vi "SlideBoundsWrite.vi"(4 "error in (no error)":errorcluster, 5 "Value":cluster{"min":i16, "max":i16}, 6 "Container State":T2, 7 "Display State In":T1) -> (0 "error out":errorcluster, 3 "Display State Out":T1)   [LabVIEW 2019, in "XVerticalSlide.xctl"]
uses:
  XVerticalSlide.xctl
  <vilib>/_xctls/Container State.ctl
  State.ctl
  <vilib>/_xctls/XControlSupport.lvlib
panel:
  # "Replace the Value Control below with a Control of desired type.\nDo not remove this Control or the others from the connector pane.\nDo not change the connector pane pattern.\nThe Value control should always be the third terminal from top on the input side in the connector pane."
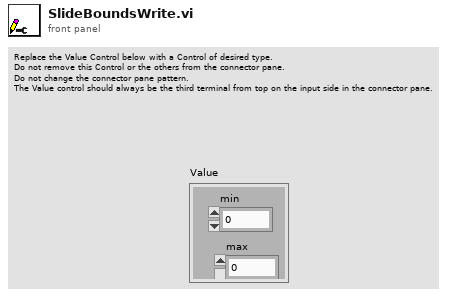
[diagram p1: front panel]
types:
  T1 = typedef "XVerticalSlide.xctl/State.ctl" = cluster{"low":i16, "high":i16, "min":i16, "max":i16}
  T2 = typedef "XControlSupport.lvlib/Container State.ctl" = cluster{"Indicator?":bool, "Run Mode?":bool, " Refnum":refnum<vi>}
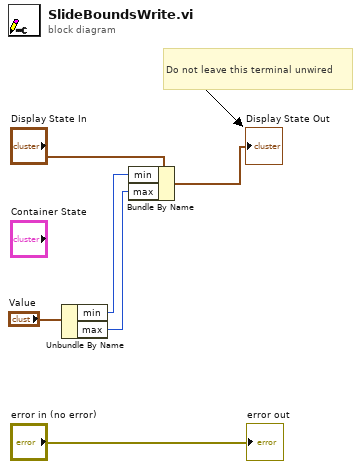
[diagram p0: block diagram]
diagram:
  # "Do not leave this terminal unwired"
  n1 = Unbundle By Name("Value") -> ("min"=w3:i16, "max"=w2:i16)
  n2 = Bundle By Name(cluster="Display State In", "min"=w3, "max"=w2) -> (→"Display State Out":T1)
  "error out" <- "error in (no error)"
